vi "Measurement Logic.vi"(8 "error in":errorcluster, 9 "measurement configuration":T2={"double in"=1.2, "Input Terminal Name"="", "DUT Pin"=""}, 10 "measure call context in":refnum<class "Measure Call Context.lvclass">) -> (0 "error out":errorcluster, 1 "measurement results":T1, 2 "measure call context out":refnum<class "Measure Call Context.lvclass">)   [LabVIEW 2025, in "Daqmx-Display.lvclass"]
doc: "Contains the core logic for executing the measurement."
uses:
  Daqmx-Display.lvclass
  Daqmx-Display.lvclass/Daqmx-Display.ctl
  Measurement Results.ctl
  <vilib>/Plug-In SDKs/Measurements/Measure Call Context/Measure Call Context.lvclass
  <vilib>/Plug-In SDKs/Clients/Session Management V1/Session Reservation/Session Reservation.lvclass
  session-management/daqmxDI/Session Management daqmxDI.lvlib
  <vilib>/DAQmx/create/channels.llb/DAQmx Create Channel (DI-Digital Input).vi
  <vilib>/DAQmx/read.llb/DAQmx Read (Digital 1D Bool 1Chan 1Samp).vi
  Measurement Configuration.ctl
panel:
  out "stop":bool
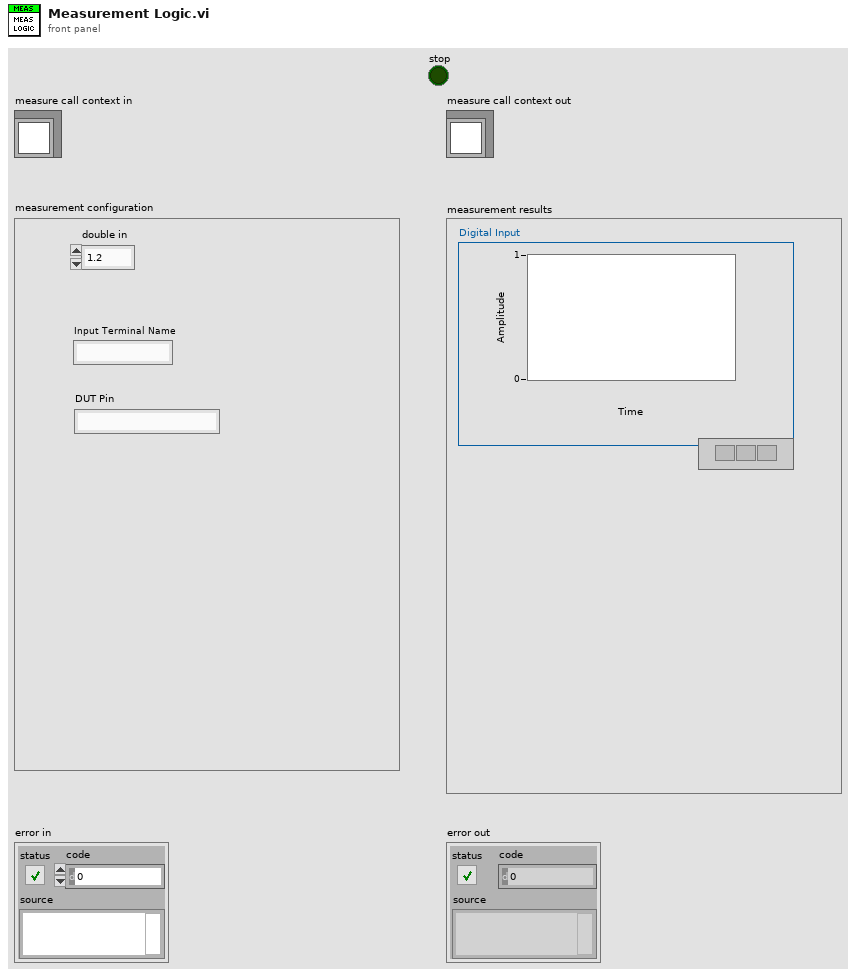
[diagram p1: front panel]
types:
  T1 = typedef "Daqmx-Display.lvclass/Measurement Results.ctl" = cluster{"Digital Input":u32[]}
  T2 = typedef "Daqmx-Display.lvclass/Measurement Configuration.ctl" = cluster{"double in":dbl, "Input Terminal Name":string, "DUT Pin":string}
  T3 = typedef "Session Management daqmxDI.lvlib/Connection with Session.ctl" = cluster{"connection":T4, "session":string}
  T4 = typedef "NI Session Management V1 Client.lvlib/Session Reservation.lvclass/Connection.ctl" = cluster{"pin or relay name":string, "site":i32, "instrument type id":string, "channel":string}
  T5 = typedef "Event Messenger-bool.lvlib/))Channel.ctl" = refnum<queue>
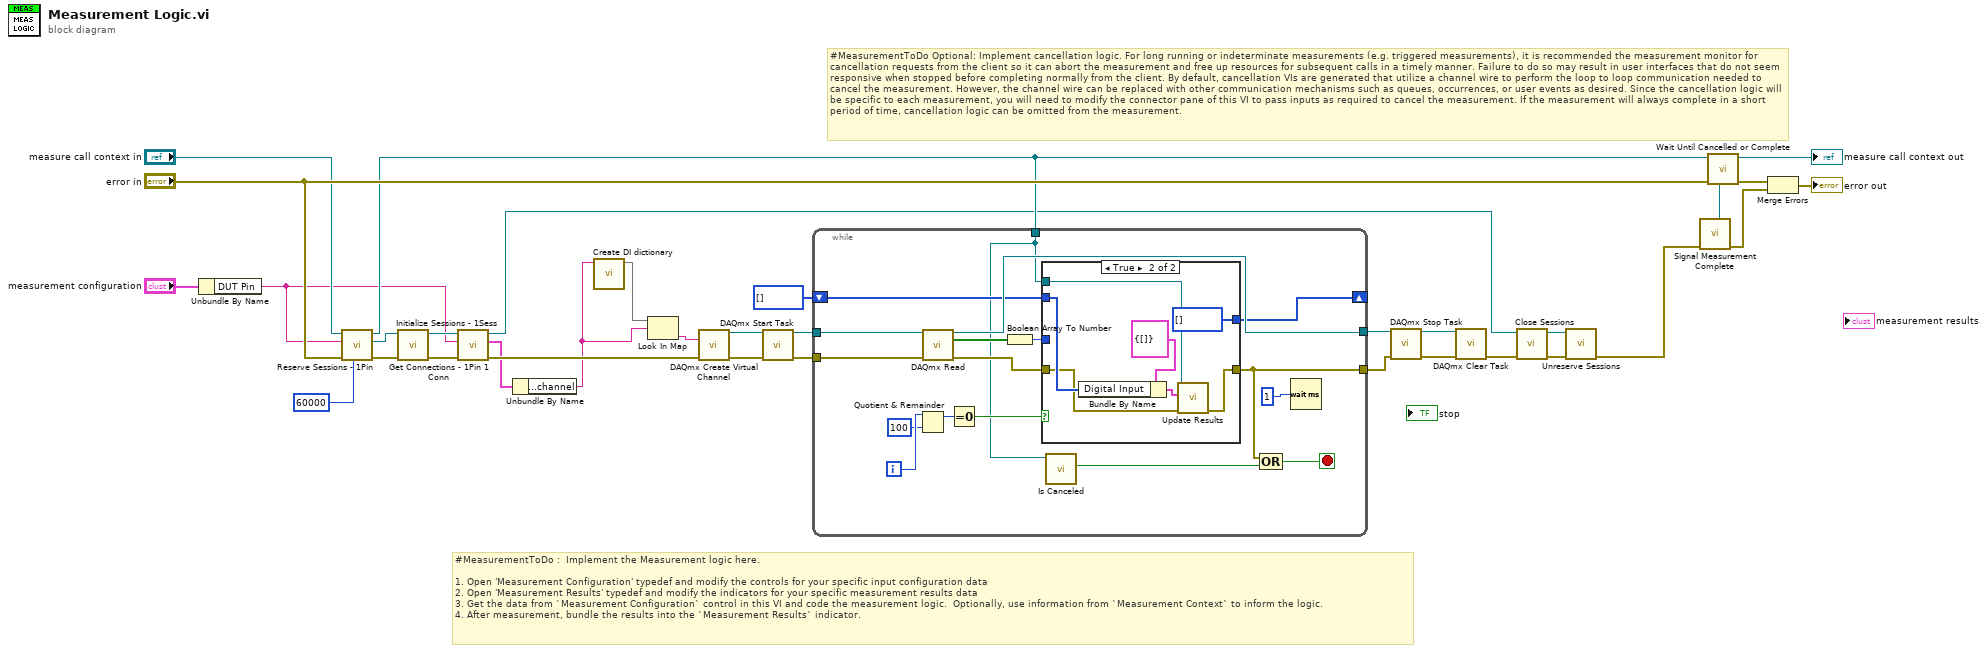
[diagram p0: block diagram]
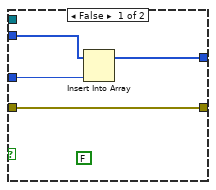
[diagram p2: hidden frame]
diagram:
  # "#MeasurementToDo Optional: Implement cancellation logic. For long running or indeterminate measurements (e.g. triggered measurements), it is recommended the measurement monitor for cancellation requests from the client so it can abort the measurement and free up resources for subsequent calls in a timely manner. Failure to do so may result in user interfaces that do not seem responsive when stopped before completing normally from the client. By default, cancellation VIs are generated that utilize a channel wire to perform the loop to loop communication needed to cancel the measurement. However, the channel wire can be replaced with other communication mechanisms such as queues, occurrences, or user events as desired. Since the cancellation logic will be specific to each measurement, you will need to modify the connector pane of this VI to pass inputs as required to cancel the measurement. If the measurement will always complete in a short period of time, cancellation logic can be omitted from the measurement."
  # "#MeasurementToDo :  Implement the Measurement logic here.\n\n1. Open 'Measurement Configuration' typedef and modify the controls for your specific input configuration data\n2. Open 'Measurement Results' typedef and modify the indicators for your specific measurement results data\n3. Get the data from `Measurement Configuration` control in this VI and code the measurement logic.  Optionally, use information from `Measurement Context` to inform the logic.\n4. After measurement, bundle the results into the `Measurement Results` indicator."
  n1 = Unbundle By Name("measurement configuration") -> ("DUT Pin"=w4:string)
  n2 = call <vilib>:"Reserve Sessions - 1Pin.vi"("timeout (ms)"=60000 ("timeout in milliseconds"), "error in"="error in", "pin or relay name"=w4, "measurement context in"="measure call context in") -> ("error out"=w12:errorcluster, "session reservation out"=w13:refnum<class "Session Reservation.lvclass">, "measurement context out"=w9:refnum<class "Measure Call Context.lvclass">)  [unwired: 5 in]
  n3 = call "Initialize Sessions - 1Sess.vi"("error in"=w12, "session reservation in"=w13) -> ("error out"=w5:errorcluster, "session reservation out"=w7:refnum<class "Session Reservation.lvclass">)  [unwired: 6 in, 2 out]
  n4 = call "Get Connections - 1Pin 1 Conn.vi"("error in"=w5, "pin or relay name"=w4, "session reservation in"=w7) -> ("error out"=w3:errorcluster, "connection"=w2:T3, "session reservation out"=w6:refnum<class "Session Reservation.lvclass">)  [unwired: 6 in]
  n5 = Unbundle By Name(w2) -> ("connection.channel"=w1:string)
  n6 = call "Create DI dictionary.vi"("PFI Input"=w1) -> ("map"=w21:map{string, string})  [unwired: 10 in]
  n7 = Look In Map(map=w21, key=w1) -> (value=w20:string)  [unwired: 1 in, 1 out]
  n8 = call-poly <vilib>:"DAQmx Create Virtual Channel.vi"("lines"=w20, "error in"=w3) -> ("task out"=w27:refnum<k21>, "error out"=w28:errorcluster)  [unwired: 12 in]
  n9 = call <vilib>:"DAQmx Start Task.vi"("task/channels in"=w27, "error in"=w28) -> ("task out"=w26:refnum<k21>, "error out"=w25:errorcluster)  [unwired: 12 in]
  n10 = while {
    tunnel: [w51] -> w22
    tunnel: w26 -> [w50]
    shift-right: [w42] -> _
    shift-left: u32[] [] -> [w41]
    tunnel: w25 -> [w39]
    tunnel: w9 -> [w36]
    tunnel: [w35] -> w8
    i -> [w48]
    stop <- w40 stop-if-true
    n11 = Quotient & Remainder(x=w48, y=100) -> (x-y*floor(x/y)=w46:i32)  [unwired: 1 out]
    n12 = call-poly <vilib>:"DAQmx Read.vi"("task/channels in"=w50, "error in"=w39) -> ("task out"=w51:refnum<k21>, "data"=w44:bool[], "error out"=w38:errorcluster)  [unwired: 11 in]
    n13 = Equal To 0?(x=w46) -> (x = 0?=w45:bool)
    n14 = Boolean Array To Number(Boolean array=w44) -> (number=w43:u32)
    n15 = case shown="True" w45 {
      tunnel: w43 -> [w54 _]
      tunnel: w41 -> [w55 w60]
      tunnel: [w53 u32[] []] -> w42
      tunnel: w38 -> [w52 w57]
      tunnel: [w52 w56] -> w35
      tunnel: w36 -> [_ w59]
      frame False {
        (unwired) FALSE ("is canceled?")
        n16 = Insert Into Array(array=w55, new element=w54) -> (w53:u32[])  [unwired: 1 in]
      }
      frame True {
        n17 = Bundle By Name(cluster=T1 {"Digital Input"=[]} ("Measurement Results"), "Digital Input"=w60) -> (w58:T1)
        n18 = call <vilib>:"Update Results.vi"("error in"=w57, "measurement results"=w58, "measure call context in"=w59) -> ("error out"=w56:errorcluster)  [unwired: 7 in, 1 out]
      }
    }
    n19 = call <vilib>:"Is Canceled.vi"("measure call context in"=w36) -> ("is canceled?"=w37:bool)  [unwired: 8 in, 2 out]
    n20 = Compound Arithmetic op=OR(w35, w37) -> (w40:bool)
    n21 = Wait (ms)(milliseconds to wait=u32 1 ("Loop Time (ms)")) -> ()  [unwired: 1 out]
  }
  n22 = call <vilib>:"DAQmx Stop Task.vi"("task/channels in"=w22, "error in"=w8) -> ("task out"=w24:refnum<k21>, "error out"=w23:errorcluster)  [unwired: 12 in]
  n23 = call <vilib>:"DAQmx Clear Task.vi"("task in"=w24, "error in"=w23) -> ("error out"=w17:errorcluster)  [unwired: 13 in]
  n24 = call <vilib>:"Close Sessions.vi"("error in"=w17, "session reservation in"=w6) -> ("error out"=w16:errorcluster, "session reservation out"=w18:refnum<class "Session Reservation.lvclass">)  [unwired: 8 in]
  n25 = call <vilib>:"Unreserve Sessions.vi"("error in"=w16, "session reservation in"=w18) -> ("error out"=w15:errorcluster)  [unwired: 9 in]
  n26 = call "Signal Measurement Complete.vi"("error in (no error)"=w15) -> ("error out"=w32:errorcluster, "done channel"=w33:T5)  [unwired: 9 in]
  n27 = call "Wait Until Cancelled or Complete.vi"("done channel"=w33, "error in (no error)"="error in", "measure call context in"=w9) -> ("error out"=w31:errorcluster, "measure call context out"=→"measure call context out":refnum<class "Measure Call Context.lvclass">)  [unwired: 7 in]
  n28 = Merge Errors(w31, w32) -> (→"error out":errorcluster)
